vi "Remove Duplicates for String Array.vi"(11 "Array in":string[](array[string])) -> (3 "Array out":string[](array[string]))   [LabVIEW 2017, in "CSM Shared.lvlib"]
uses:
  CSM Shared.lvlib
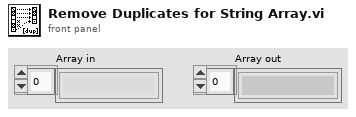
[diagram p1: front panel]
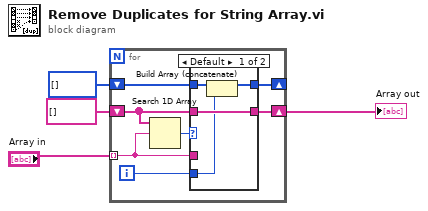
[diagram p0: block diagram]
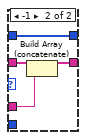
[diagram p2: hidden frame]
diagram:
  n1 = for {
    tunnel: "Array in" -> [w10] mode=indexing
    shift-right: [w9] -> w1
    shift-left: string[] [] -> [w8]
    shift-right: [w6] -> _
    shift-left: i32[] [] -> [w5]
    i -> [w7]
    n2 = Search 1D Array(1D array=w8, element=w10) -> (index of element=w11:i32)  [unwired: 1 in]
    n3 = case shown="Default" w11 {
      tunnel: w10 -> [_ w19]
      tunnel: [w15 w17] -> w9
      tunnel: w8 -> [w15 w18]
      tunnel: w7 -> [w12 _]
      tunnel: [w13 w16] -> w6
      tunnel: w5 -> [w14 w16]
      frame Default {
        n4 = Build Array (concatenate)(w14, w12) -> (w13:i32[])
      }
      frame -1 {
        n5 = Build Array (concatenate)(w18, w19) -> (w17:string[])
      }
    }
  }
  "Array out" <- w1
